vi "run_embedding_core.vi"(0 "llm_openai_embedding in":refnum<class "llm_openai_embedding.lvclass">, 5 "data":refnum<class "abstract_message_base.lvclass">[](array[class]), 11 "error in (no error)":errorcluster) -> (4 "llm_openai_embedding out":refnum<class "llm_openai_embedding.lvclass">, 6 "embedding response":refnum<class "message_vectors.lvclass">[](array[class]), 15 "error out":errorcluster)   [LabVIEW 2020, in "llm_openai_embedding.lvclass"]
uses:
  llm_openai_embedding.lvclass
  abstract_message_base/abstract_message_base.lvclass
  message_vectors/message_vectors.lvclass
  <vilib>/NI/Progress Bar/Controls/Progress Bar Properties.ctl
  <vilib>/NI/Progress Bar/Controls/Update Bar Actions.ctl
  <vilib>/httpClient/POSTBuffer.vi
  <vilib>/httpClient/LabVIEWHTTPClient.lvlib
  <vilib>/NI/Progress Bar/Progress Bar.lvlib
panel:
  out "body":string
  out "headers":string
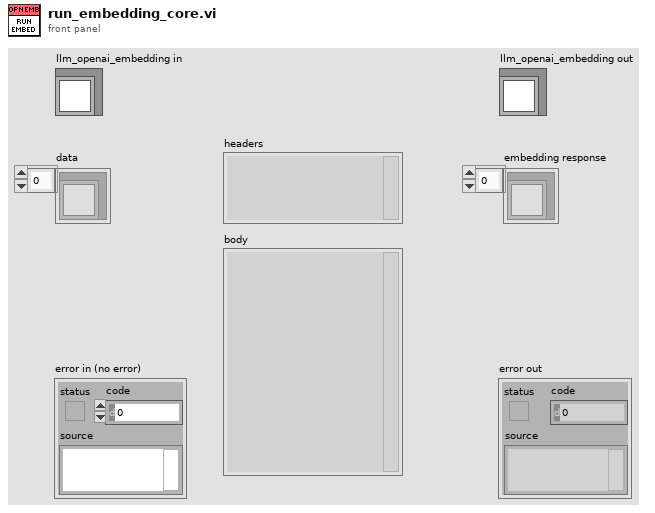
[diagram p1: front panel]
types:
  T1 = typedef "Progress Bar.lvlib/Update Bar Actions.ctl" = enum16{"Add To Existing", "Set to Value"}
  T2 = typedef "Progress Bar.lvlib/Progress Bar Properties.ctl" = cluster{"Background Color":u32, "Installer Title":string, "Title Color":u32, "Action Text":string, "Text Color":u32, "Slider Value":u8, "Bar Color":u32, "Timeout":i32}
  T3 = typedef "LabVIEWHTTPClient.lvlib/ClientHandle.ctl" = refnum<k1>
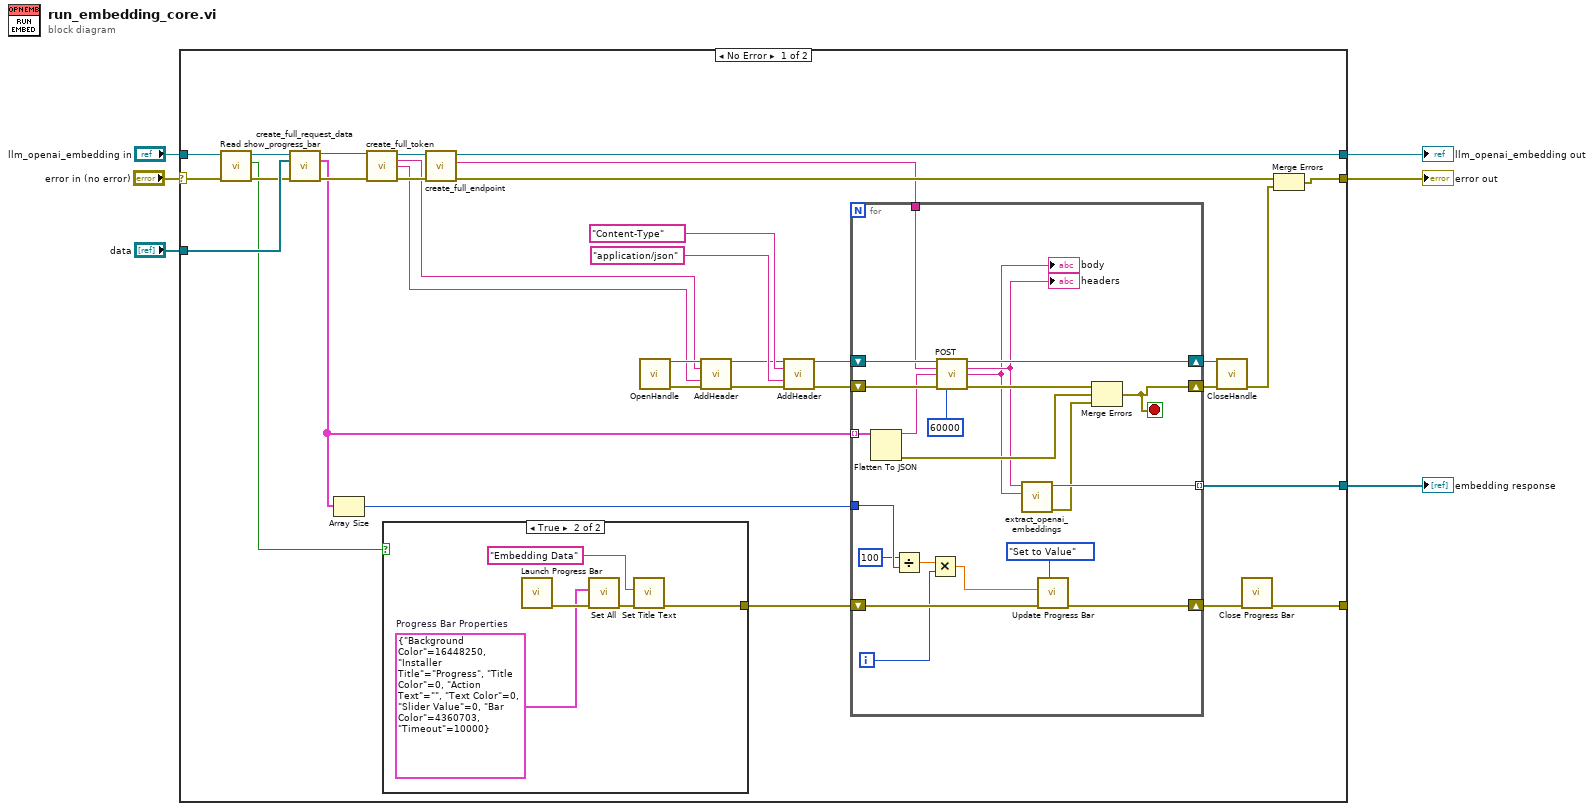
[diagram p0: block diagram]
diagram:
  n1 = case shown="No Error" "error in (no error)" {
    selector: "error in (no error)" -> [w9 w68]
    tunnel: [w19 w68] -> w5
    tunnel: [w28 w67] -> w4
    tunnel: "llm_openai_embedding in" -> [w11 w67]
    tunnel: "data" -> [w21 _]
    tunnel: [w17 _] -> w1
    tunnel: [w13 _] -> _
    frame No Error {
      n2 = call-dynamic "Read show_progress_bar.vi"("error in (no error)"=w9, "abstract_llm_base in"=w11) -> ("error out"=w8:errorcluster, "show_progress_bar"=w7:bool, "abstract_llm_base out"=w10:refnum<class "llm_openai_embedding.lvclass">)  [unwired: 7 in]
      n3 = call-dynamic "create_full_request_data.vi"("llm_openai_embedding in"=w10, "data"=w21, "error in (no error)"=w8) -> ("llm_openai_embedding out"=w22:refnum<class "llm_openai_embedding.lvclass">, "request_data"=w15:cluster{"input":string, "model":string}[], "error out"=w23:errorcluster)  [unwired: 10 in]
      n4 = Array Size(array=w15) -> (size(s)=w12:i32)
      n5 = call-dynamic "create_full_token.vi"("llm_openai_embedding in"=w22, "error in (no error)"=w23) -> ("llm_openai_embedding out"=w29:refnum<class "llm_openai_embedding.lvclass">, "header"=w25:string, "token"=w24:string, "error out"=w30:errorcluster)  [unwired: 10 in]
      n6 = case shown="True" w7 {
        tunnel: [_ w40] -> w16
        frame False {
        }
        frame True {
          w41 = T2 {"Background Color"=16448250, "Installer Title"="Progress", "Title Color"=0, "Action Text"="", "Text Color"=0, "Slider Value"=0, "Bar Color"=4360703, "Timeout"=10000}  # Progress Bar Properties
          n7 = call <vilib>:"Launch Progress Bar.vi"() -> ("error out"=w42:errorcluster)  [unwired: 10 in, 1 out]
          n8 = call <vilib>:"Set All.vi"("error in (no error)"=w42, "Progress Bar Properties (Default)"=w41) -> ("error out"=w43:errorcluster)  [unwired: 9 in]
          n9 = call <vilib>:"Set Title Text.vi"("error in (no error)"=w43, "Installer Title"="Embedding Data") -> ("error out"=w40:errorcluster)  [unwired: 9 in]
        }
      }
      n10 = call-dynamic "create_full_endpoint.vi"("error in (no error)"=w30, "llm_openai_embedding in"=w29) -> ("error out"=w27:errorcluster, "endpoint"=w26:string, "llm_openai_embedding out"=w28:refnum<class "llm_openai_embedding.lvclass">)  [unwired: 7 in]
      n11 = call <vilib>:"OpenHandle.vi"() -> ("client handle out"=w39:T3, "error out"=w38:errorcluster)  [unwired: 14 in]
      n12 = call <vilib>:"AddHeader.vi"("client handle"=w39, "header"=w25, "value"=w24, "error in (no error)"=w38) -> ("client handle out"=w35:T3, "error out"=w33:errorcluster)  [unwired: 10 in]
      n13 = call <vilib>:"AddHeader.vi"("client handle"=w35, "header"="Content-Type", "value"="application/json", "error in (no error)"=w33) -> ("client handle out"=w34:T3, "error out"=w32:errorcluster)  [unwired: 10 in]
      n14 = for {
        tunnel: w26 -> [w62]
        shift-right: [w64] -> w31
        shift-left: w34 -> [w66]
        tunnel: w15 -> [w60] mode=indexing
        shift-right: [w57] -> w20
        shift-left: w32 -> [w65]
        tunnel: [w54] -> w17 mode=indexing
        shift-right: [w51] -> w14
        shift-left: w16 -> [w52]
        tunnel: w12 -> [w49]
        i -> [w46]
        stop <- w57 stop-if-true
        n15 = Flatten To JSON(anything=w60) -> (JSON string=w59:string, 11:w58:errorcluster)  [unwired: 2 in]
        n16 = Divide(x=100, y=w49) -> (x/y=w47:dbl)
        n17 = Multiply(x=w47, y=w46) -> (x*y=w45:dbl)
        n18 = call-poly <vilib>:"POST.vi"("client handle"=w66, "url"=w62, "buffer"=w59, "error in (no error)"=w65, "timeout (10000)"=60000) -> ("client handle out"=w64:T3, "headers"=w56:string, "body"=w55:string, "error out"=w61:errorcluster)  [unwired: 7 in]
        "headers" <- w56
        "body" <- w55
        n19 = call "extract_openai_embeddings.vi"("body"=w55, "headers"=w56) -> ("error out"=w53:errorcluster, "vector response"=w54:refnum<class "message_vectors.lvclass">)  [unwired: 8 in]
        n20 = call <vilib>:"Update Progress Bar.vi"("Action"=Update_Bar_Actions."Set to Value", "error in (no error)"=w52, "Value"=w45) -> ("error out"=w51:errorcluster)  [unwired: 8 in]
        n21 = Merge Errors(w61, w58, w53) -> (w57:errorcluster)
      }
      n22 = call <vilib>:"CloseHandle.vi"("client handle"=w31, "error in (no error)"=w20) -> ("error out"=w18:errorcluster)  [unwired: 13 in]
      n23 = call <vilib>:"Close Progress Bar.vi"("error in (no error)"=w14) -> ("error out"=w13:errorcluster)  [unwired: 9 in, 1 out]
      n24 = Merge Errors(w27, w18) -> (w19:errorcluster)
    }
    frame Error {
    }
  }
  "error out" <- w5
  "llm_openai_embedding out" <- w4
  "embedding response" <- w1
